vi "CheckUserPass.vi"(7 "ConnectionString":string, 8 "error in":errorcluster, 9 "password":string, 10 "user":string, 11 "connection ID in":refnum<k5>) -> (0 "error out":errorcluster, 1 "endtime":string, 2 "starttime":string, 3 "connection ID out":refnum<k5>, 4 "id":string, 5 "result":bool, 6 "error out sql":errorcluster)   [LabVIEW 2010]
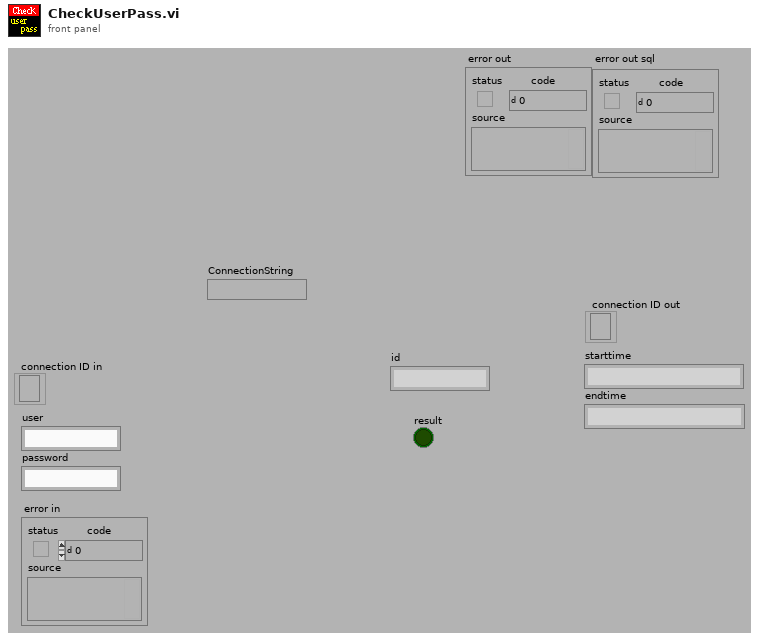
[diagram p1: front panel]
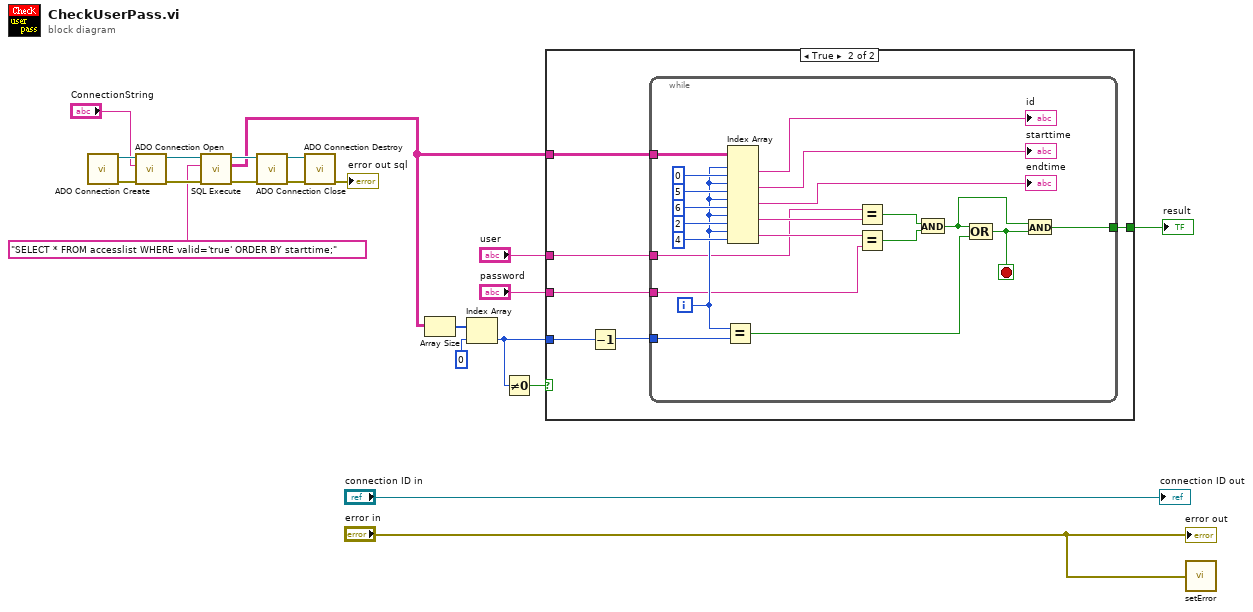
[diagram p0: block diagram]
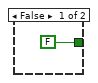
[diagram p2: hidden frame]
diagram:
  n1 = call "ADO Connection Create.vi"() -> ("error out"=w13:errorcluster, "ADODB._Connection Out"=w12:refnum<k7>)  [unwired: 1 in, 9 out]
  n2 = call "ADO Connection Open.vi"("error in (no error)"=w13, "ConnectionString"="ConnectionString", "ADODB._Connection In"=w12) -> ("error out"=w8:errorcluster, "ADODB._Connection Out"=w9:refnum<k7>)  [unwired: 7 out]
  n3 = call "SQL Execute.vi"("error in (no error)"=w8, "Command Text"="SELECT * FROM accesslist WHERE valid='true' ORDER BY starttime;", "ADODB._Connection In"=w9) -> ("error out"=w7:errorcluster, "Data"=w5:string[][], "ADODB._Connection Out"=w6:refnum<k7>)  [unwired: 1 in, 5 out]
  n4 = call "ADO Connection Close.vi"("error in (no error)"=w7, "ADODB._Connection In"=w6) -> ("error out"=w11:errorcluster, "ADODB._Connection Out"=w10:refnum<k7>)  [unwired: 8 out]
  n5 = call "ADO Connection Destroy.vi"("error in (no error)"=w11, "ADODB._Connection In"=w10) -> ("error out"=→"error out sql":errorcluster)  [unwired: 9 out]
  n6 = Array Size(array=w5) -> (size(s)=w21:i32[])
  n7 = Index Array(array=w21, index=0) -> (element=w14:i32)
  n8 = Not Equal To 0?(x=w14) -> (x != 0?=w15:bool)
  n9 = case shown="True" w15 {
    tunnel: w14 -> [_ w28]
    tunnel: w5 -> [_ w27]
    tunnel: [FALSE w25] -> w18
    tunnel: "user" -> [_ w24]
    tunnel: "password" -> [_ w23]
    frame False {
    }
    frame True {
      n10 = Decrement(x=w28) -> (x-1=w26:i32)
      n11 = while {
        tunnel: w27 -> [w49]
        tunnel: w26 -> [w42]
        tunnel: w24 -> [w34]
        tunnel: w23 -> [w33]
        tunnel: [w32] -> w25
        i -> [w43]
        stop <- w35 stop-if-true
        n12 = Equal?(x=w43, y=w42) -> (x = y?=w37:bool)
        n13 = Index Array(array=w49, index (row) #1=w43, index (col) #1=0 ("disabled index (col)"), index (row) #2=w43, index (col) #2=5 ("disabled index (col)"), index (row) #3=w43, index (col) #3=6 ("disabled index (col)"), index (row) #4=w43, index (col) #4=2 ("disabled index (col)"), index (row) #5=w43, index (col) #5=4 ("disabled index (col)")) -> (element #1=→"id":string, element #2=→"starttime":string, element #3=→"endtime":string, element #4=w41:string, element #5=w40:string)
        n14 = Equal?(x=w34, y=w41) -> (x = y?=w39:bool)
        n15 = Equal?(x=w40, y=w33) -> (x = y?=w38:bool)
        n16 = And(x=w39, y=w38) -> (x .and. y?=w36:bool)
        n17 = Compound Arithmetic op=OR(w36, w37) -> (w35:bool)
        n18 = And(x=w36, y=w35) -> (x .and. y?=w32:bool)
      }
    }
  }
  "result" <- w18
  n19 = call "setError.vi"("error"="error in") -> ()  [unwired: 1 out]
  "connection ID out" <- "connection ID in"
  "error out" <- "error in"
